vi "email_worker.vi"(8 "error in (no error)":errorcluster) -> (0 "error out":errorcluster)   [LabVIEW 2020]
panel:
  out "loops":i32
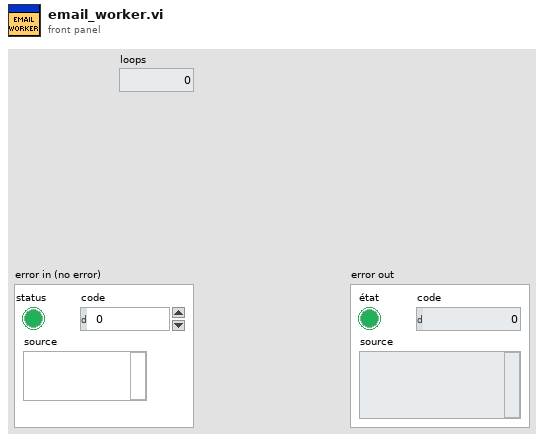
[diagram p1: front panel]
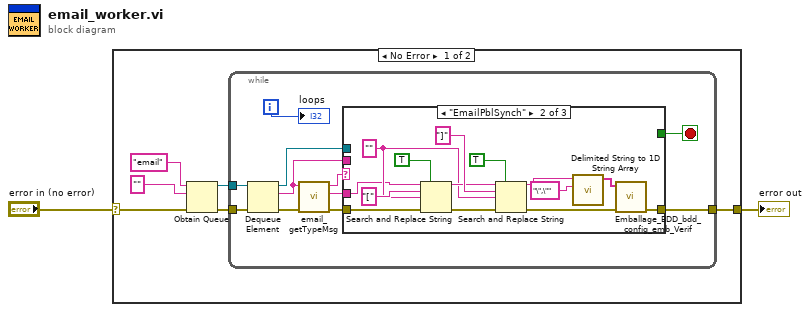
[diagram p0: block diagram]
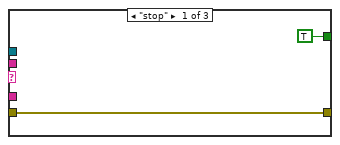
[diagram p2: hidden frame]
diagram:
  n1 = case shown="No Error" "error in (no error)" {
    selector: "error in (no error)" -> [w3 w37]
    tunnel: [w8 w37] -> w1
    frame No Error {
      n2 = Obtain Queue(name (unnamed)="email" ("nom (aucun)"), element data type="" ("nom (aucun)"), error in (no error)=w3) -> (queue out=w4:refnum<queue>, error out=w5:errorcluster)  [unwired: 2 in, 1 out]
      n3 = while {
        tunnel: [w19] -> w8
        tunnel: w5 -> [w17]
        tunnel: w4 -> [w16]
        i -> [w15]
        stop <- w18 stop-if-true
        n4 = Dequeue Element(queue=w16, error in (no error)=w17) -> (queue out=w14:refnum<queue>, element=w11:string, error out=w13:errorcluster)  [unwired: 1 in, 1 out]
        n5 = call "email_getTypeMsg.vi"("entrée d'erreur (pas d'erreur)"=w13, "trimmed string"=w11) -> ("sortie d'erreur"=w12:errorcluster, "content"=w9:string, "typeMsg"=w10:string)  [unwired: 7 in]
        n6 = case shown="\"EmailPblSynch\"" w10 {
          tunnel: [w21 w35 w36] -> w19
          tunnel: w12 -> [w21 w22 w36]
          tunnel: [TRUE ("Stop?") _ _] -> w18
          tunnel: w11 -> [_ _ _]
          tunnel: w14 -> [_ _ _]
          tunnel: w9 -> [_ w24 _]
          frame "stop" {
          }
          frame "EmailPblSynch" {
            w25 = "" ("replace string (\"\")")
            n7 = Search and Replace String(replace all?=TRUE ("replace all? (F)"), input string=w24, search string="[", replace string=w25, error in=w22) -> (result string=w32:string, error out=w27:errorcluster)  [unwired: 3 in, 2 out]
            n8 = Search and Replace String(replace all?=TRUE ("replace all? (F)"), input string=w32, search string="]", replace string=w25, error in=w27) -> (result string=w29:string, error out=w26:errorcluster)  [unwired: 3 in, 2 out]
            n9 = call <vilib>:"Delimited String to 1D String Array.vi"("delimiter"="\",\"", "delimited string"=w29) -> ("string array"=w23:string[])  [unwired: 9 in]
            n10 = call "Emballage_BDD_bdd_config_emb_Verif.vi"("Error in"=w26, "tableau_config"=w23) -> ("Error out"=w35:errorcluster)  [unwired: 9 in]
          }
          frame "na", Default {
          }
        }
        "loops" <- w15
      }
    }
    frame Error {
    }
  }
  "error out" <- w1
